vi "togle.vi"(2 "Boolean 3":bool) -> (7 "Boolean 4":bool)   [LabVIEW 2018]
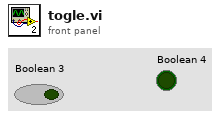
[diagram p1: front panel]
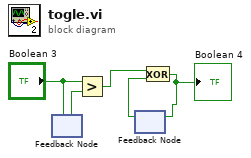
[diagram p0: block diagram]
diagram:
  n1 = feedback #1() -> (w2:bool)  [unwired: 1 in]
  n2 = feedback-in #1("Boolean 3") -> ()
  n3 = Greater?(x="Boolean 3", y=w2) -> (0:w5:bool)
  n4 = feedback #2() -> (w3:bool)  [unwired: 1 in]
  n5 = Exclusive Or(1:w3, 2:w5) -> (0:w4:bool)
  "Boolean 4" <- w4
  n6 = feedback-in #2(w4) -> ()
